vi "Valid Path.vi"(1 "Path":path) -> (0 "Valid":bool)   [LabVIEW 2015]
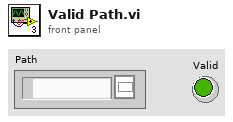
[diagram p1: front panel]
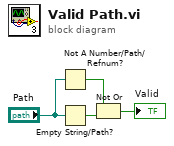
[diagram p0: block diagram]
diagram:
  n1 = Not A Number/Path/Refnum?(number/path/refnum="Path") -> (NaN/Path/Refnum?=w3:bool)
  n2 = Empty String/Path?(string/path="Path") -> (empty?=w4:bool)
  n3 = Not Or(1:w4, 2:w3) -> (0:→"Valid":bool)
